vi "Start Sequence Acquisition.vi"(8 "error in (no error)":errorcluster, 11 "DAQ_QPT_Throlab in":refnum<class "DAQ_QPT_Throlab.lvclass">) -> (0 "error out":errorcluster, 3 "DAQ_QPT_Throlab out":refnum<class "DAQ_QPT_Throlab.lvclass">)   [LabVIEW 2020, in "DAQ_QPT_Throlab.lvlib" / "DAQ_QPT_Throlab.lvclass"]
uses:
  DAQ_QPT_Throlab.lvclass
  Hardware Abstraction Layer/Component/DAQ/DAQ/DAQ.lvclass
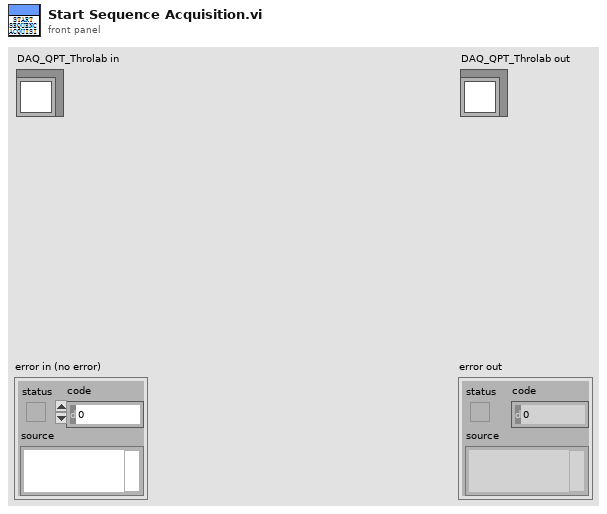
[diagram p1: front panel]
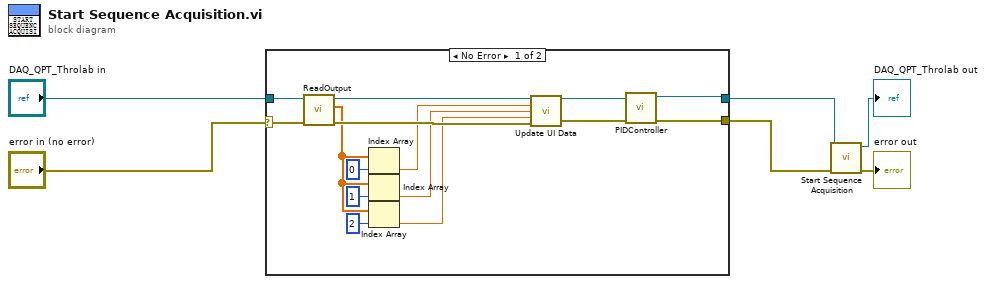
[diagram p0: block diagram]
diagram:
  n1 = case shown="No Error" "error in (no error)" {
    selector: "error in (no error)" -> [w20 w22]
    tunnel: "DAQ_QPT_Throlab in" -> [w21 w23]
    tunnel: [w9 w22] -> w3
    tunnel: [w7 w23] -> w1
    frame No Error {
      n2 = call-dynamic "ReadOutput.vi"("error in (no error)"=w20, "DAQ_QPT_Throlab in"=w21) -> ("error out"=w18:errorcluster, "Output Values"=w16:dbl[], "DAQ_QPT_Throlab out"=w19:refnum<class "DAQ_QPT_Throlab.lvclass">)  [unwired: 7 in]
      n3 = Index Array(array=w16, index=0) -> (element=w12:dbl)
      n4 = Index Array(array=w16, index=1) -> (element=w11:dbl)
      n5 = Index Array(array=w16, index=2) -> (element=w10:dbl)
      n6 = call-dynamic "Update UI Data.vi"("DAQ in"=w19, "QPD Voltage X"=w12, "QPD Voltage Y"=w11, "QPD  Sum"=w10, "error in (no error)"=w18) -> ("DAQ out"=w8:refnum<class "DAQ_QPT_Throlab.lvclass">, "error out"=w17:errorcluster)  [unwired: 9 in]
      n7 = call-dynamic "PIDController.vi"("error in (no error)"=w17, "DAQ_QPT_Throlab in"=w8) -> ("error out"=w9:errorcluster, "DAQ_QPT_Throlab out"=w7:refnum<class "DAQ_QPT_Throlab.lvclass">)  [unwired: 8 in]
    }
    frame Error {
    }
  }
  n8 = call-parent "Start Sequence Acquisition.vi"("error in (no error)"=w3, "DAQ in"=w1) -> ("error out"=→"error out":errorcluster, "DAQ out"=→"DAQ_QPT_Throlab out":refnum<class "DAQ_QPT_Throlab.lvclass">)  [unwired: 8 in]
